vi "setBurstState.vi"(8 "error in (no error)":errorcluster, 10 "State":bool, 11 "VISA resource name":refnum<visa-resource-name>) -> (0 "error out":errorcluster, 3 "VISA resource name out":refnum<visa-resource-name>)   [LabVIEW 2023, in "Keysight-33500B.lvlib"]
doc: "<b>Author:</b> Wolfgang\n<b>Description:</b>\nEnables or disables burst mode.\nOutput phase is set to 0 when burst is enabled.\nl To avoid multiple waveform changes, enable the burst mode after configuring the other burst parameters.\nl The instrument will not allow the burst mode to be enabled at the same time that sweep or any modulation mode is enabled. When you enable burst, the sweep or modulation mode is turned off."
uses:
  Keysight-33500B.lvlib
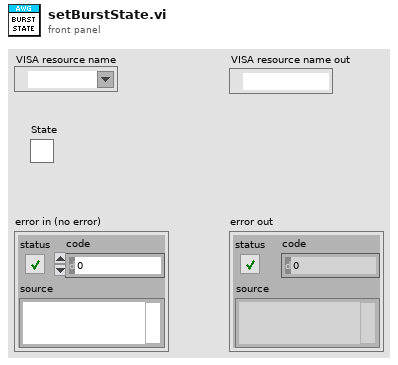
[diagram p1: front panel]
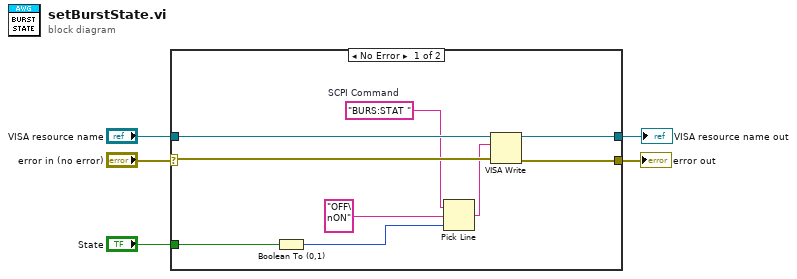
[diagram p0: block diagram]
diagram:
  n1 = case shown="No Error" "error in (no error)" {
    selector: "error in (no error)" -> [w11 w16]
    tunnel: [w13 w15] -> w5
    tunnel: [w14 w16] -> w3
    tunnel: "VISA resource name" -> [w12 w15]
    tunnel: "State" -> [w10 _]
    frame No Error {
      w9 = "BURS:STAT "  # SCPI Command
      n2 = Boolean To (0,1)(Boolean=w10) -> (0, 1=w6:i16)
      n3 = Pick Line(string ("")=w9, multi-line string="OFF\nON" ("format string"), line index=w6) -> (output string=w8:string)
      n4 = VISA Write(VISA resource name=w12, write buffer=w8, error in (no error)=w11) -> (VISA resource name out=w13:refnum<visa-resource-name>, error out=w14:errorcluster)  [unwired: 1 out]
    }
    frame Error {
    }
  }
  "VISA resource name out" <- w5
  "error out" <- w3
